vi "readrems2.vi"() -> ()   [LabVIEW 2010]
doc: "Пакетный режим выполнения вишек."
uses:
  <vilib>/Utility/miscctls.llb/LVRectTypeDef.ctl
panel:
  out "String":string
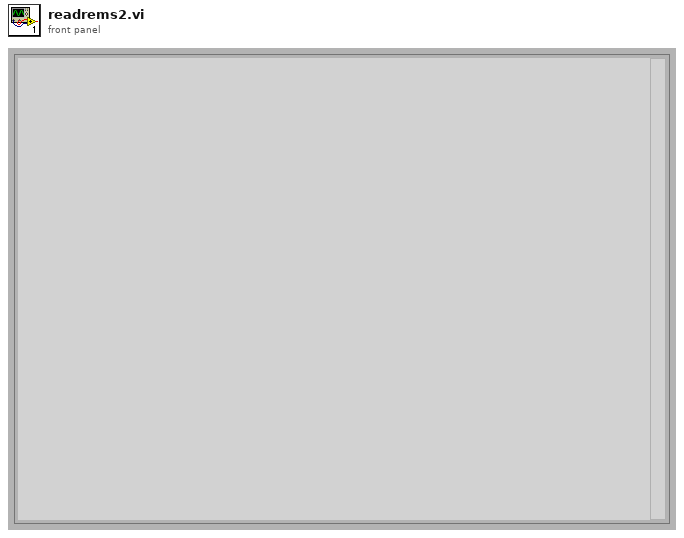
[diagram p1: front panel]
types:
  T1 = typedef "LVRectTypeDef.ctl" = cluster{"Left":i16, "Top":i16, "Right":i16, "Bottom":i16}
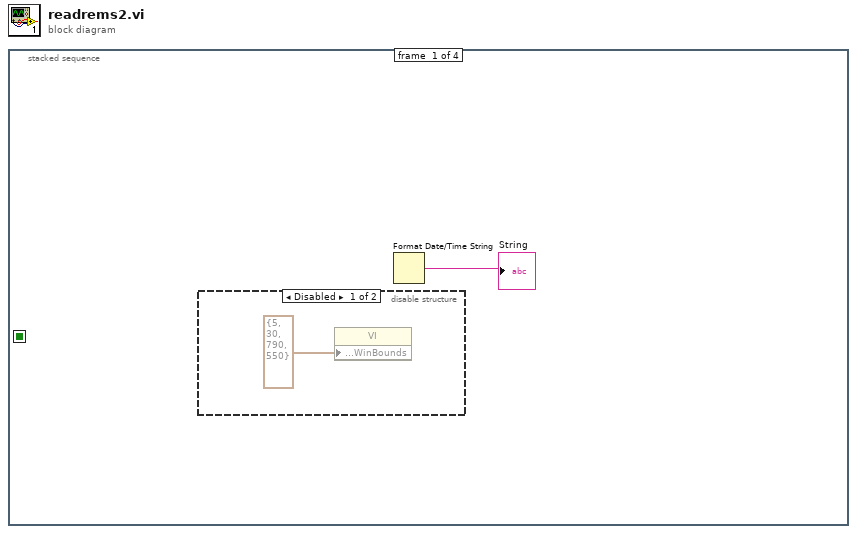
[diagram p0: block diagram]
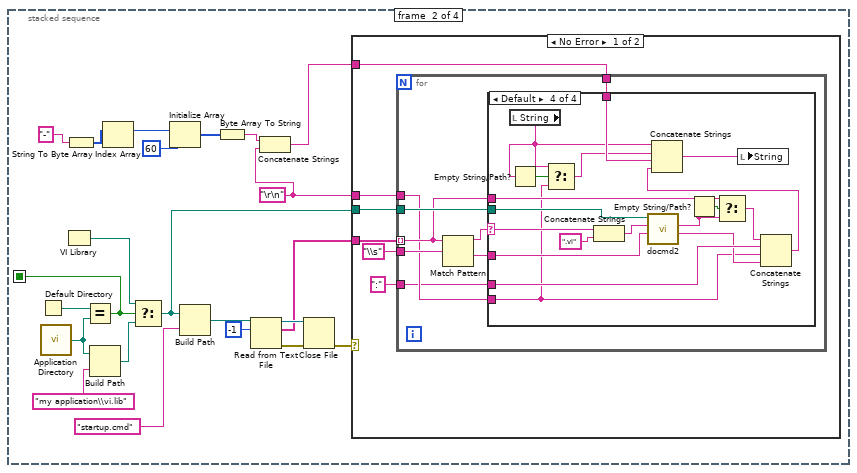
[diagram p3: hidden frame]
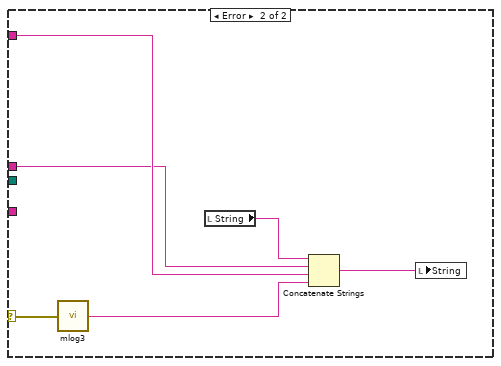
[diagram p7: hidden frame]
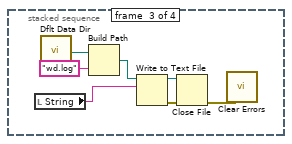
[diagram p8: hidden frame]
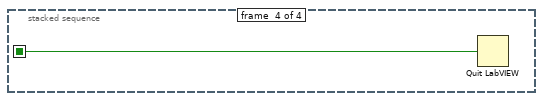
[diagram p9: hidden frame]
diagram:
  n1 = stacked-sequence {
    seq-local: [_ w4 _ _] -> [_ _ _ w70]
    frame #0 {
      n2 = disable-structure shown="Disabled" {
        frame Disabled {
          n3 = property class="VI"("Front Panel.WinBounds"=T1 {"Left"=5, "Top"=30, "Right"=790, "Bottom"=550} ("Front Panel Window:Window Bounds")) -> ()  [unwired: 2 in, 2 out]
        }
        frame Enabled {
        }
      }
      n4 = Format Date/Time String() -> (date/time string=→"String":string)  [unwired: 3 in]
    }
    frame #1 {
      w6 = "\r\n"
      n5 = Default Directory() -> (w20:path)
      n6 = call <vilib>:"Application Directory.vi"() -> ("Application Directory"=w19:path)
      n7 = VI Library() -> (path=w23:path)
      n8 = String To Byte Array(string="-") -> (unsigned byte array=w9:u8[])
      n9 = Equal?(x=w20, y=w19) -> (x = y?=w4:bool)
      n10 = Build Path(base path=w19, name or relative path="my application\\vi.lib") -> (appended path=w18:path)
      n11 = Index Array(array=w9) -> (element=w8:u8)  [unwired: 1 in]
      n12 = Select(t=w23, s=w4, f=w18) -> (s? t:f=w13:path)
      n13 = Initialize Array(w8, 60 ("dimension size")) -> (w12:u8[])
      n14 = Build Path(base path=w13, name or relative path="startup.cmd") -> (appended path=w3:path)
      n15 = Byte Array To String(unsigned byte array=w12) -> (string=w7:string)
      n16 = Read from Text File(file (use dialog)=w3, count=-1) -> (refnum out=w22:refnum<file>, text=w14:string[], error out=w21:errorcluster)  [unwired: 2 in, 1 out]
      n17 = Concatenate Strings(w7, w6) -> (w5:string)
      n18 = Close File(refnum=w22, error in=w21) -> (error out=w15:errorcluster)  [unwired: 1 out]
      n19 = case shown="No Error" w15 {
        selector: w15 -> [_ w62]
        tunnel: w14 -> [w30 _]
        tunnel: w13 -> [w29 _]
        tunnel: w6 -> [w28 w57]
        tunnel: w5 -> [w27 w59]
        frame No Error {
          n20 = for {
            tunnel: w30 -> [w35] mode=indexing
            tunnel: w29 -> [w38]
            tunnel: w28 -> [w33]
            tunnel: "\\s" ("regular expression") -> [w34]
            tunnel: ":" ("string") -> [w32]
            tunnel: w27 -> [w31]
            n21 = Match Pattern(string=w35, regular expression=w34) -> (before substring=w36:string, after substring=w37:string)  [unwired: 1 in, 2 out]
            n22 = case shown="Default" w36 {
              selector: w36 -> [_ _ _ w52]
              tunnel: w38 -> [_ _ _ w56]
              tunnel: w37 -> [_ _ _ w55]
              tunnel: w35 -> [_ _ _ w49]
              tunnel: w33 -> [_ _ _ w41]
              tunnel: w32 -> [_ _ _ w47]
              tunnel: w31 -> [_ _ _ w45]
              frame "rem" {
              }
              frame ";" {
              }
              frame "%" {
              }
              frame Default {
                n23 = local read "String"() -> (w40:string)
                n24 = Empty String/Path?(string/path=w40) -> (empty?=w42:bool)
                n25 = Select(t=w40, s=w42, f=w41) -> (s? t:f=w39:string)
                n26 = Concatenate Strings(w52, ".vi" ("string")) -> (w53:string)
                n27 = call "docmd2.vi"("Param"=w55, "VI_Name"=w53, "CMDpath"=w56) -> ("rezult"=w46:string, "VI Description"=w50:string)  [unwired: 3 in]
                n28 = Empty String/Path?(string/path=w50) -> (empty?=w51:bool)
                n29 = Select(t=w49, s=w51, f=w50) -> (s? t:f=w48:string)
                n30 = Concatenate Strings(w48, w47, w41, w46) -> (w44:string)
                n31 = Concatenate Strings(w40, w39, w45, w44) -> (w43:string)
                n32 = local write "String"(w43) -> ()
              }
            }
          }
        }
        frame Error {
          n33 = call "mlog3.vi"("error in"=w62) -> ("message"=w58:string)
          n34 = local read "String"() -> (w61:string)
          n35 = Concatenate Strings(w61, w57, w59, w58) -> (w60:string)
          n36 = local write "String"(w60) -> ()
        }
      }
    }
    frame #2 {
      n37 = local read "String"() -> (w63:string)
      n38 = call <vilib>:"Dflt Data Dir.vi"() -> ("App:Default Data Directory"=w66:path)
      n39 = Build Path(base path=w66, name or relative path="wd.log") -> (appended path=w67:path)
      n40 = Write to Text File(file (use dialog)=w67, text=w63) -> (refnum out=w64:refnum<file>, error out=w68:errorcluster)  [unwired: 2 in, 1 out]
      n41 = Close File(refnum=w64, error in=w68) -> (error out=w69:errorcluster)  [unwired: 1 out]
      n42 = call <vilib>:"Clear Errors.vi"("error in (no error)"=w69) -> ()  [unwired: 6 in, 1 out]
    }
    frame #3 {
      n43 = Quit LabVIEW(quit? (T)=w70) -> ()
    }
  }
